vi "Queue Actor.vi"(6 "Creator":refnum<data-value>, 8 "Creator Alias":string, 9 "Self Alias":string, 10 "Queue of Queue Self":refnum<queue>, 11 "Queue jettl":refnum<class "Queue jettl.lvclass">) -> ()   [LabVIEW 2021, in "jettl.lvlib" / "Base Queue jettl.lvlib" / "Base Queue jettl.lvclass"]
uses:
  Base Queue jettl.lvclass
  Base Queue jettl.lvclass/Base Queue jettl.ctl
  jettl.lvlib
  Queue jettl/Queue jettl.lvclass
  Queue Last Ack/Queue Last Ack.lvlib
  Msg Strategy/Msg Strategy.lvclass
  C:/git/jettl/src/jettl/jettl/jettl.lvclass
  C:/git/jettl/src/jettl/Merge Error/Merge Error/Merge Error.lvclass
  C:/git/jettl/src/jettl/Queue jettl/Queue jettl.lvclass
  C:/git/jettl/src/jettl/Event Create/Event Create/Event Create.lvclass
  C:/git/jettl/src/jettl/Event Last Ack/Event Last Ack/Event Last Ack.lvclass
  C:/git/jettl/src/jettl/Override Error/Override Error/Override Error.lvclass
  C:/git/jettl/src/jettl/Queue Create/Queue Create/Queue Create.lvclass
  C:/git/jettl/src/jettl/Queue Last Ack/Queue Last Ack/Queue Last Ack.lvclass
  C:/git/jettl/src/jettl/Setup/Setup/Setup.lvclass
  C:/git/jettl/src/jettl/Teardown/Teardown/Teardown.lvclass
  C:/git/jettl/src/jettl/Base Queue jettl/Base Queue jettl/Base Queue jettl.lvclass
  Queue Last Ack/Queue Last Ack Msg Strategy/Queue Last Ack Msg Strategy.lvclass
  C:/git/jettl/src/jettl/Queue Last Ack/Queue Last Ack Msg Strategy/Queue Last Ack Msg Strategy.lvclass
  C:/git/jettl/src/jettl/Msg Strategy/Msg Strategy.lvclass
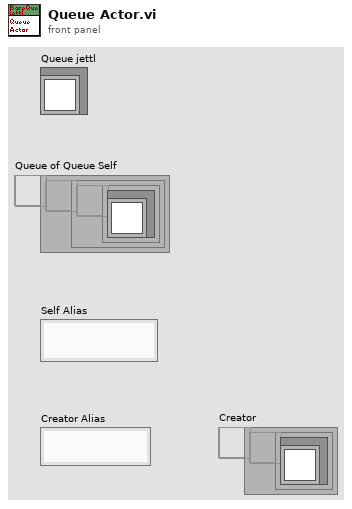
[diagram p1: front panel]
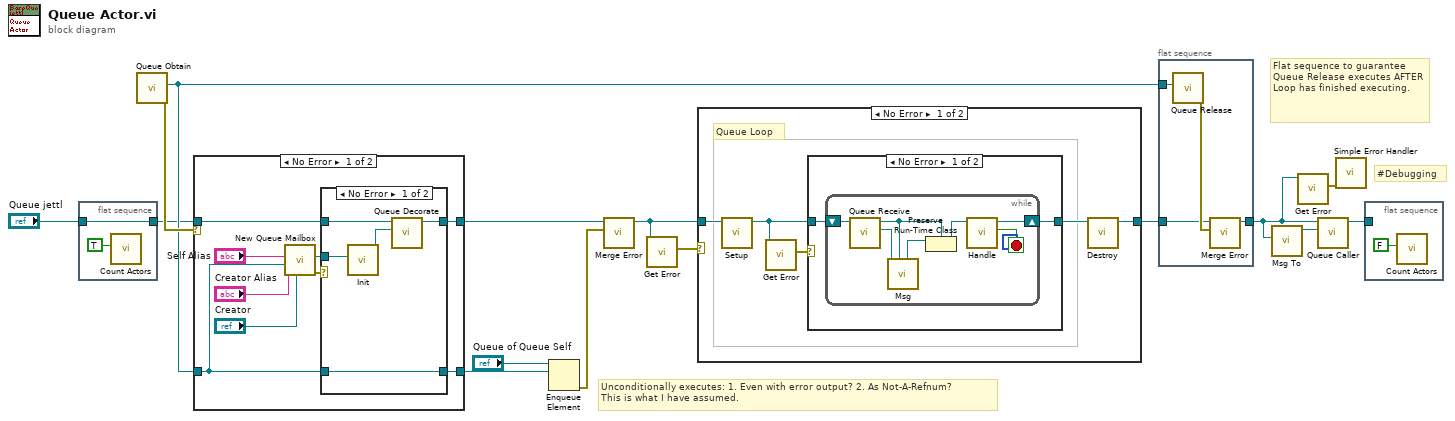
[diagram p0: block diagram]
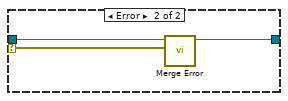
[diagram p3: hidden frame]
diagram:
  # "#Debugging"
  # "Flat sequence to guarantee Queue Release executes AFTER Loop has finished executing."
  # "Unconditionally executes: 1. Even with error output? 2. As Not-A-Refnum?\nThis is what I have assumed."
  n1 = flat-sequence {
    tunnel: [w16] -> w5
    tunnel: "Queue jettl" -> [w16]
    frame #0 {
      n2 = call "Count Actors.vi"("Increment?"=TRUE) -> ()  [unwired: 11 in]
    }
  }
  n3 = call "Queue Obtain.vi"() -> ("error out"=w15:errorcluster, "Queue"=w12:refnum<data-value>)  [unwired: 10 in]
  n4 = case shown="No Error" w15 {
    selector: w15 -> [_ w34]
    tunnel: [w25 w35] -> w11
    tunnel: w5 -> [w26 w33]
    tunnel: w12 -> [w18 _]
    tunnel: [w23 _] -> w10
    frame No Error {
      n5 = call "New Queue Mailbox.vi"("Creator"="Creator", "Creator Alias"="Creator Alias", "Self"=w18, "Self Alias"="Self Alias") -> ("error out"=w22:errorcluster, "Queue Mailbox"=w24:refnum<data-value>)  [unwired: 6 in]
      n6 = case shown="No Error" w22 {
        tunnel: w26 -> [w31 w32]
        tunnel: [w29 w32] -> w25
        tunnel: w24 -> [w28 _]
        tunnel: [w27 _] -> w23
        tunnel: w18 -> [w27 _]
        frame No Error {
          n7 = call "Init.vi"("Queue Mailbox"=w28) -> ("Base Queue jettl out"=w30:refnum<class "Base Queue jettl.lvclass">)  [unwired: 10 in]
          n8 = call-dynamic "Queue Decorate.vi"("Queue jettl"=w30, "Queue jettl in"=w31) -> ("Queue jettl out"=w29:refnum<class "Queue jettl.lvclass">)  [unwired: 9 in]
        }
        frame Error {
        }
      }
    }
    frame Error {
      n9 = call-dynamic "Merge Error.vi"("Error"=w34, "Merge Error in"=w33) -> ("Merge Error out"=w35:refnum<class "Queue jettl.lvclass">)  [unwired: 9 in]
    }
  }
  n10 = Enqueue Element(queue="Queue of Queue Self", element=w10) -> (error out=w13:errorcluster)  [unwired: 2 in, 2 out]
  n11 = call-dynamic "Merge Error.vi"("Error"=w13, "Merge Error in"=w11) -> ("Merge Error out"=w14:refnum<class "Queue jettl.lvclass">)  [unwired: 9 in]
  n12 = call-dynamic "Get Error.vi"("jettl in"=w14) -> ("Error"=w9:errorcluster)  [unwired: 10 in]
  n13 = case shown="No Error" w9 {
    tunnel: w14 -> [w38 w51]
    tunnel: [w39 w51] -> w8
    frame No Error {
      # "Queue Loop"
      n14 = call-dynamic "Setup.vi"("Setup in"=w38) -> ("Setup out"=w36:refnum<class "Queue jettl.lvclass">)  [unwired: 10 in]
      n15 = call-dynamic "Get Error.vi"("jettl in"=w36) -> ("Error"=w37:errorcluster)  [unwired: 10 in]
      n16 = case shown="No Error" w37 {
        tunnel: [w42 w50] -> w40
        tunnel: w36 -> [w41 w50]
        frame No Error {
          n17 = while "Queue Loop" {
            shift-right: [w49] -> w42
            shift-left: w41 -> [w48]
            stop <- w46 stop-if-true
            n18 = call-dynamic "Queue Receive.vi"("Queue jettl in"=w48) -> ("Msg Strategy"=w47:refnum<class "Msg Strategy.lvclass">, "Queue jettl out"=w45:refnum<class "Queue jettl.lvclass">)  [unwired: 9 in]
            n19 = call-dynamic "Msg.vi"("jettl in"=w45, "Msg Strategy in"=w47) -> ("jettl out"=w43:refnum<class "jettl.lvclass">)  [unwired: 9 in]
            n20 = Preserve Run-Time Class(object in=w43, 2:w45) -> (object out=w44:refnum<class "Queue jettl.lvclass">)  [unwired: 1 in, 1 out]
            n21 = call-dynamic "Handle.vi"("jettl in"=w44) -> ("Destroy?"=w46:bool, "jettl out"=w49:refnum<class "Queue jettl.lvclass">)  [unwired: 9 in]
          }
        }
        frame Error {
        }
      }
      n22 = call-dynamic "Destroy.vi"("jettl in"=w40) -> ("jettl out"=w39:refnum<class "Queue jettl.lvclass">)  [unwired: 10 in]
    }
    frame Error {
    }
  }
  n23 = flat-sequence {
    tunnel: w12 -> [w55]
    tunnel: [w54] -> w2
    tunnel: w8 -> [w52]
    frame #0 {
      n24 = call "Queue Release.vi"("Queue"=w55) -> ("error out"=w53:errorcluster)  [unwired: 10 in]
      n25 = call-dynamic "Merge Error.vi"("Error"=w53, "Merge Error in"=w52) -> ("Merge Error out"=w54:refnum<class "Queue jettl.lvclass">)  [unwired: 9 in]
    }
  }
  n26 = call "Msg To.vi"("Queue jettl"=w2) -> ("Queue Last Ack Msg Strategy out"=w3:refnum<class "Queue Last Ack Msg Strategy.lvclass">)  [unwired: 10 in]
  n27 = call-dynamic "Get Error.vi"("jettl in"=w2) -> ("Error"=w7:errorcluster)  [unwired: 10 in]
  n28 = call-dynamic "Queue Caller.vi"("Msg Strategy"=w3, "jettl in"=w2) -> ("jettl out"=w4:refnum<class "Queue jettl.lvclass">)  [unwired: 9 in]
  n29 = call <vilib>:"Simple Error Handler.vi"("error in (no error)"=w7) -> ()  [unwired: 4 in, 5 out]
  n30 = flat-sequence {
    tunnel: w4 -> [_]
    frame #0 {
      n31 = call "Count Actors.vi"("Increment?"=FALSE) -> ()  [unwired: 11 in]
    }
  }
